vi "UART Read.vi"   [LabVIEW 2014, in "LMH-LINX.lvlib"]
uses:
  <vilib>/MakerHub/LINX/LMH-LINX.lvlib
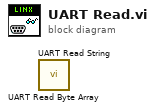
[diagram p0: block diagram]
diagram:
  n1 = call <vilib>:"UART Read Byte Array.vi"() -> ()  [unwired: 9 in, 3 out]
  n2 = call <vilib>:"UART Read String.vi"() -> ()  [unwired: 9 in, 3 out]
